vi "lv stream buffer.vi"(8 "error in":errorcluster, 10 "size per ch":u32, 11 "channels":i32[](array[numeric])) -> (0 "error out":errorcluster, 3 "buffer handle":i32)   [LabVIEW 2026]
uses:
  bin/nominalClient_64.dll
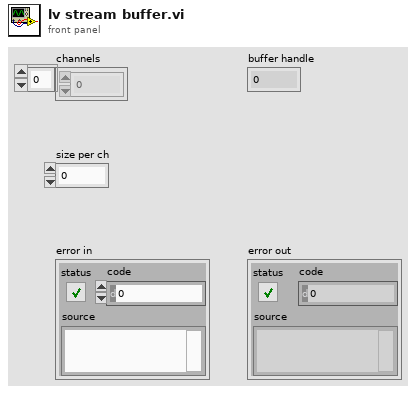
[diagram p1: front panel]
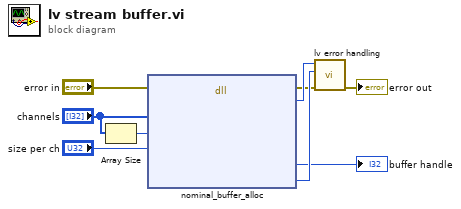
[diagram p0: block diagram]
diagram:
  n1 = Array Size(array="channels") -> (size(s)=w2:i32)
  n2 = dll-call lib="C:/sw/nominal-c/bin/nominalClient_64.dll" fn="nominal_buffer_alloc"(error in="error in", "channels"="channels", "channel count"=w2, "capacity"="size per ch") -> (error out=w6:errorcluster, "return type"=w7:i32, "buffer handle"=→"buffer handle":i32, "errorout"=w8:i32)  [unwired: 7 in, 1 out]
  n3 = call "lv error handling.vi"("error in"=w6, "error handle"=w8, "return code"=w7) -> ("error out"=→"error out":errorcluster)  [unwired: 8 in]
